vi "Robot Main.vi"   [LabVIEW 2011]
doc: "This VI imlements the framework and scheduler for your robotics program. It should not be necessary to modify the framework. You are expected to add your code to the VIs called from Robot Main, the ones located in the Team Code within the project."
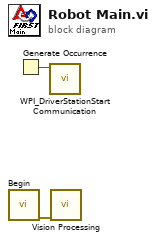
[diagram p0: block diagram]
diagram:
  n1 = call "Begin.vi"() -> ("error out"=w1:errorcluster)  [unwired: 1 in, 10 out]
  n2 = Generate Occurrence() -> (w2:refnum<k4>)
  n3 = call <vilib>:"WPI_DriverStationStart Communication.vi"("occurrence"=w2) -> ()  [unwired: 11 out]
  n4 = call "Vision Processing.vi"("error in (no error)"=w1) -> ()  [unwired: 1 in, 6 out]
